vi "GCMPlugin_GetPluginName.vi"(8 "error in (no error)":errorcluster, 11 "TemplatePlugin in":refnum<class "EXESpecEditor.lvclass">) -> (0 "error out":errorcluster, 2 "PluginName":string, 3 "TemplatePlugin out":refnum<class "EXESpecEditor.lvclass">)   [LabVIEW 2014, in "BuildSpecEditor.lvlib" / "EXESpecEditor.lvclass"]
uses:
  EXESpecEditor.lvclass
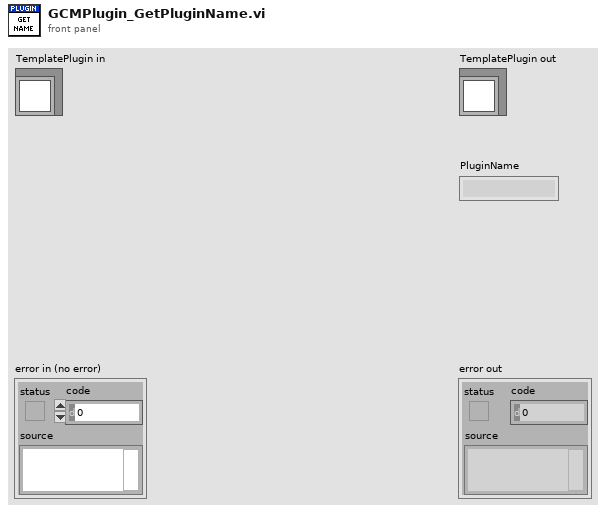
[diagram p1: front panel]
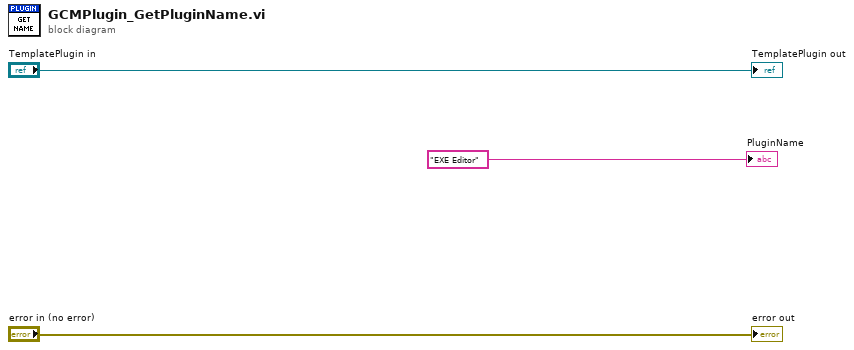
[diagram p0: block diagram]
diagram:
  "error out" <- "error in (no error)"
  "TemplatePlugin out" <- "TemplatePlugin in"
  "PluginName" <- "EXE Editor"
